vi "Determine Distance to Tags from all Tags.vi"(0 "Input TagsArray":refnum<class "Tag.lvclass">[](array[class]), 5 "DistanceLimitTag":dbl=70.0, 7 "Enable Error margin?":bool, 9 "Error Margin":dbl=2.0, 12 "error in (no error)":errorcluster) -> (6 "AllTagDistancesArray":T1(array[cluster]), 10 "AltTDA":T1(array[cluster]), 14 "error out":errorcluster)   [LabVIEW 2014]
doc: "This VI calculates the distance between all Tags."
uses:
  Tag.lvclass
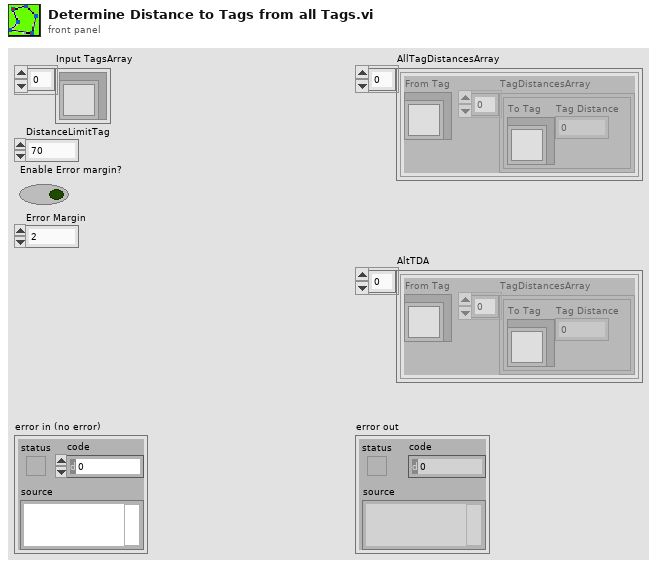
[diagram p1: front panel]
types:
  T1 = cluster{"From Tag":refnum<class "Tag.lvclass">, "TagDistancesArray":cluster{"To Tag":refnum<class "Tag.lvclass">, "Tag Distance":dbl}[]}[]
  T2 = cluster{"From Tag":refnum<class "Tag.lvclass">, "TagDistancesArray":cluster{"To Tag":refnum<class "Tag.lvclass">, "Tag Distance":dbl}[]}
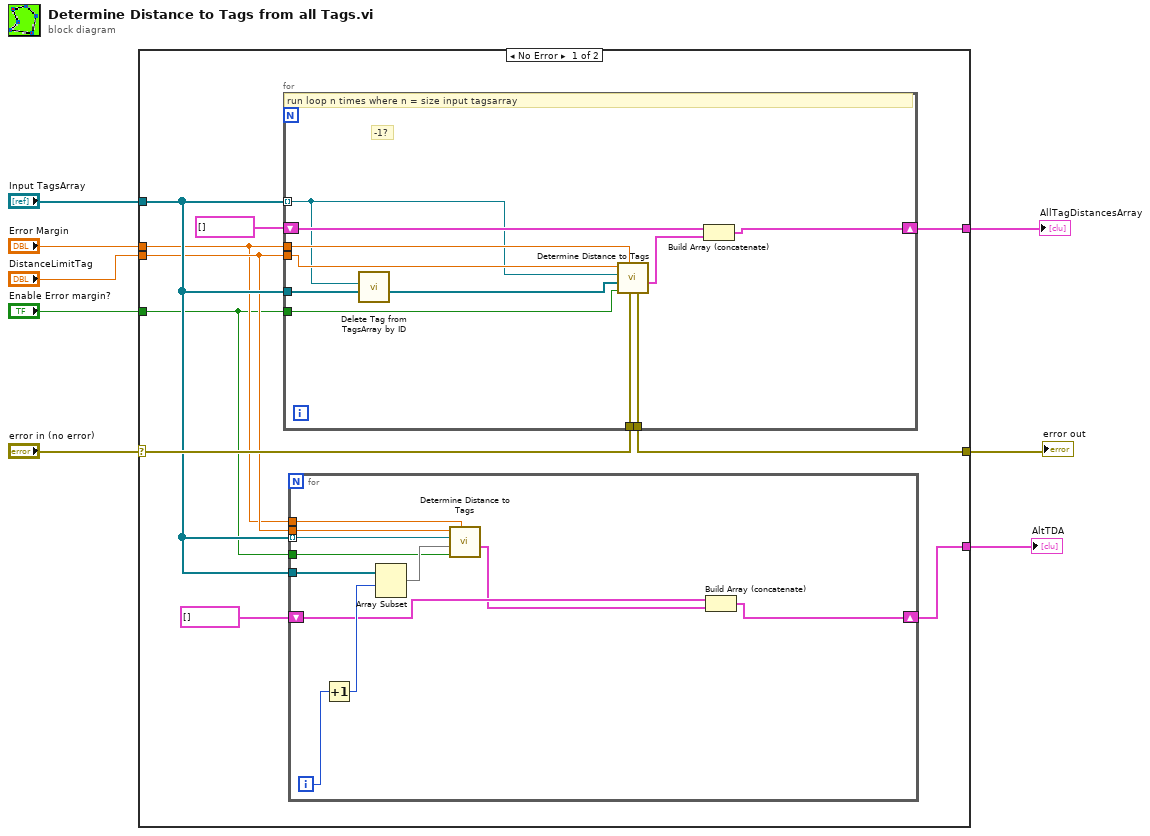
[diagram p0: block diagram]
diagram:
  n1 = case shown="No Error" "error in (no error)" {
    selector: "error in (no error)" -> [w18 w41]
    tunnel: [w17 w41] -> w7
    tunnel: "Input TagsArray" -> [w14 _]
    tunnel: "Error Margin" -> [w12 _]
    tunnel: "DistanceLimitTag" -> [w13 _]
    tunnel: "Enable Error margin?" -> [w11 _]
    tunnel: [w15 _] -> w2
    tunnel: [w10 _] -> w1
    frame No Error {
      n2 = for {
        shift-right: [w39] -> w15
        shift-left: T1 [] -> [w40]
        tunnel: w14 -> [w33]
        tunnel: w12 -> [w38]
        tunnel: w13 -> [w37]
        tunnel: w18 -> [w36]
        tunnel: [w35] -> w17
        tunnel: w11 -> [w34]
        tunnel: w14 -> [w32] mode=indexing
        # "-1?"
        # "run loop n times where n = size input tagsarray"
        n3 = call "Delete Tag from TagsArray by ID.vi"("Input TagsArray"=w33, "Tag.lvclass"=w32) -> ("Output TagsArray"=w31:refnum<class "Tag.lvclass">[])  [unwired: 9 in]
        n4 = call "Determine Distance to Tags.vi"("error in (no error)"=w36, "Error Margin"=w38, "Enable Error margin?"=w34, "Input TagsArray"=w31, "Input Tag.lvclass"=w32, "DistanceLimitTag"=w37) -> ("TagDistancesCluster"=w30:T2, "error out"=w35:errorcluster)  [unwired: 4 in]
        n5 = Build Array (concatenate)(w40, w30) -> (w39:T1)
      }
      n6 = for {
        tunnel: w14 -> [w29] mode=indexing
        tunnel: w14 -> [w26]
        tunnel: w13 -> [w24]
        tunnel: w12 -> [w23]
        tunnel: w11 -> [w22]
        shift-right: [w21] -> w10
        shift-left: T1 [] ("AltTDA") -> [w20]
        i -> [w28]
        n7 = Increment(x=w28) -> (x+1=w27:i32)
        n8 = Array Subset(array=w26, index=w27) -> (w25:refnum<class "Tag.lvclass">[])  [unwired: 1 in]
        n9 = call "Determine Distance to Tags.vi"("Error Margin"=w23, "Enable Error margin?"=w22, "Input TagsArray"=w25, "Input Tag.lvclass"=w29, "DistanceLimitTag"=w24) -> ("TagDistancesCluster"=w19:T2)  [unwired: 5 in, 1 out]
        n10 = Build Array (concatenate)(w20, w19) -> (w21:T1)
      }
    }
    frame Error {
    }
  }
  "error out" <- w7
  "AllTagDistancesArray" <- w2
  "AltTDA" <- w1
